vi "Initialize.vi"(8 "error in (no error)":errorcluster, 11 "State in":T1={"State"=enum."Idle", "Start Time"=timestamp(0 s since 1904-01-01), "Configuration"={"Cycle Period"=0.0, "Ismatech"={"VISA resource name"="", "Simulated?"=FALSE, "Pump Number"=1.0, "Reverse?"=FALSE}, "Masterflex"={"VISA resource name"="", "Simulated?"=FALSE, "Pump Number"=1.0, "Reverse?"=FALSE}, "Manual Entry"=0.0, "VICI Settings"={"VISA resource name"="", "Simulated?"=FALSE, "Pump Letter"="", "Reverse?"=FALSE}, "Output Device"=enum."Ismatec ISM 831C", "Tacmina Settings"={"Analog DAQ Task"="", "Digital DAQ Task"=""}, "KNF SIMDOS Settings"={"VISA resource name"="", "Simulated?"=TRUE}, "ASIA Pump C"={"ASIA Pump #"=0, "channel"=0, "Simulated"=FALSE}, "FLOM Settings"={"VISA resource name"="", "Simulated?"=TRUE, "Pump Number"=0.0}, "Pump Calibration File"=path "", "Calibration Slope"=0.0, "Calibration Y Intercept"=0.0, "Pump Cal Enum"=0, "SSI PR Settings"={"VISA resource name"="", "Simulated?"=FALSE}}, "Current Time"=timestamp(0 s since 1904-01-01), "First Iteration"=FALSE, "Data"={"Pump Speed"=0.0, "Pump Pressure"=0.0, "Pump Flow"=0.0}, "Process Name"="", "Pump On?"=enum."Off", "Output Error"=FALSE, "Log Started"=FALSE, "Overpressure Alarming"=FALSE} {"Configuration"."ASIA Pump C"."channel" min=0 max=1 step=1; "Configuration"."Masterflex"."Pump Number" min=1.0 max=20.0 step=1.0; "Configuration"."Ismatech"."Pump Number" min=1.0 max=20.0 step=1.0}) -> (0 "error out":errorcluster, 1 "Initialized":bool, 3 "State out":T1={"State"=enum."Idle", "Start Time"=timestamp(0 s since 1904-01-01), "Configuration"={"Cycle Period"=0.0, "Ismatech"={"VISA resource name"="", "Simulated?"=FALSE, "Pump Number"=1.0, "Reverse?"=FALSE}, "Masterflex"={"VISA resource name"="", "Simulated?"=FALSE, "Pump Number"=1.0, "Reverse?"=FALSE}, "Manual Entry"=0.0, "VICI Settings"={"VISA resource name"="", "Simulated?"=FALSE, "Pump Letter"="", "Reverse?"=FALSE}, "Output Device"=enum."Ismatec ISM 831C", "Tacmina Settings"={"Analog DAQ Task"="", "Digital DAQ Task"=""}, "KNF SIMDOS Settings"={"VISA resource name"="", "Simulated?"=TRUE}, "ASIA Pump C"={"ASIA Pump #"=0, "channel"=0, "Simulated"=FALSE}, "FLOM Settings"={"VISA resource name"="", "Simulated?"=TRUE, "Pump Number"=0.0}, "Pump Calibration File"=path "", "Calibration Slope"=0.0, "Calibration Y Intercept"=0.0, "Pump Cal Enum"=0, "SSI PR Settings"={"VISA resource name"="", "Simulated?"=FALSE}}, "Current Time"=timestamp(0 s since 1904-01-01), "First Iteration"=FALSE, "Data"={"Pump Speed"=0.0, "Pump Pressure"=0.0, "Pump Flow"=0.0}, "Process Name"="", "Pump On?"=enum."Off", "Output Error"=FALSE, "Log Started"=FALSE, "Overpressure Alarming"=FALSE} {"Configuration"."ASIA Pump C"."channel" min=0 max=1 step=1; "Configuration"."Masterflex"."Pump Number" min=1.0 max=20.0 step=1.0; "Configuration"."Ismatech"."Pump Number" min=1.0 max=20.0 step=1.0})   [LabVIEW 2018, in "Pump Module.lvlib" / "Pump Module Engine.lvlib"]
uses:
  Pump Module Engine.lvlib
  State Cluster.ctl
  State Enum.ctl
  Pump Module Settings Cluster.ctl
  Ismatec ISM 831C/Controls/Ismatech Settings Cluster.ctl
  Masterflex 7550-30/Controls/Settings Cluster.ctl
  VICI M50 Party Mode/Settings Cluster.ctl
  Measure Instrument/PID 2 Output Enum.ctl
  Tacmina QI/Tacmina QI DAQ Setting.ctl
  KNF Pump/Settings Cluster plus SIMDOS.ctl
  ASIA Pump/Pump Settings.ctl
  FLOM Pump/Settings Cluster.ctl
  SSI PR Class/SSI PR Settings Cluster.ctl
  Tag VIs/Tag FGV Operation Enum.ctl
  Shared Variables/Dynamic Shared Variables.lvlib
  SSI PR Class/SSI PR Pump.lvlib
  FLOM Pump/FLOM Pump.lvlib
  ASIA Pump.lvlib
  KNF Pump/KNF SIMDOS.lvlib
  Tacmina QI/Tacmina QI.lvlib
  VICI M50 Party Mode/VICI M6 M50 Party Mode.lvlib
  Ismatec ISM 831C/Ismatec ISM 831C.lvlib
  Masterflex 7550-30/Masterflex 7550-30.lvlib
  Pump Module.lvlib
panel:
  # "Output Instruments"
  # "Output Instruments"
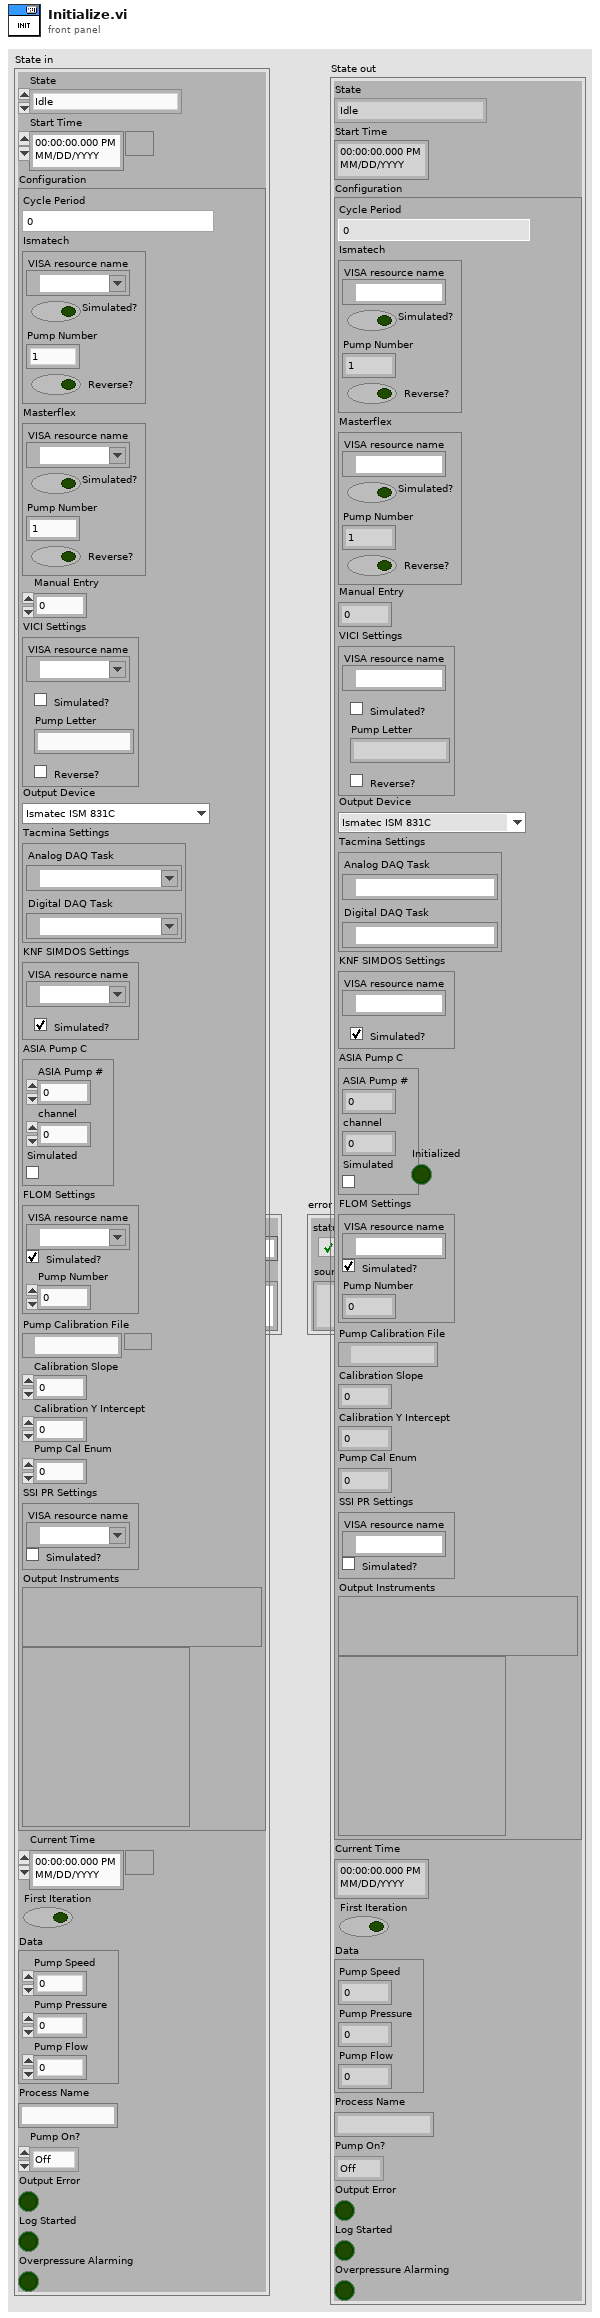
[diagram p1: front panel]
types:
  T1 = typedef "Pump Module.lvlib/Pump Module Engine.lvlib/State Cluster.ctl" = cluster{"State":T2, "Start Time":timestamp, "Configuration":T3, "Current Time":timestamp, "First Iteration":bool, "Data":cluster{"Pump Speed":dbl, "Pump Pressure":dbl, "Pump Flow":dbl}, "Process Name":string, "Pump On?":enum16{"Off", "On", "Not Initialized"}, "Output Error":bool, "Log Started":bool, "Overpressure Alarming":bool}
  T2 = typedef "Pump Module.lvlib/Pump Module Engine.lvlib/State Enum.ctl" = enum16{"Measuring", "Idle", "Paused"}
  T3 = typedef "Pump Module.lvlib/Pump Module Settings Cluster.ctl" = cluster{"Cycle Period":dbl, "Ismatech":T4, "Masterflex":T5, "Manual Entry":dbl, "VICI Settings":T6, "Output Device":T7, "Tacmina Settings":T8, "KNF SIMDOS Settings":T9, "ASIA Pump C":T10, "FLOM Settings":T11, "Pump Calibration File":path, "Calibration Slope":dbl, "Calibration Y Intercept":dbl, "Pump Cal Enum":u16, "SSI PR Settings":T12}
  T4 = typedef "Ismatec ISM 831C.lvlib/Ismatech Settings Cluster.ctl" = cluster{"VISA resource name":refnum<visa-resource-name>, "Simulated?":bool, "Pump Number":dbl, "Reverse?":bool}
  T5 = typedef "Masterflex 7550-30.lvlib/Settings Cluster.ctl" = cluster{"VISA resource name":refnum<visa-resource-name>, "Simulated?":bool, "Pump Number":dbl, "Reverse?":bool}
  T6 = typedef "VICI M6 M50 Party Mode.lvlib/Settings Cluster.ctl" = cluster{"VISA resource name":refnum<visa-resource-name>, "Simulated?":bool, "Pump Letter":string, "Reverse?":bool}
  T7 = typedef "PID 2 Output Enum.ctl" = enum16{"Default", "Ismatec ISM 831C", "Masterflex 7550-30", "VICI", "Tacmina QI", "KNF SIMDOS", "ASIA Type C", "FLOM UI-22-11", "SSI PR"}
  T8 = typedef "Tacmina QI.lvlib/Tacmina QI DAQ Setting.ctl" = cluster{"Analog DAQ Task":refnum<k21>, "Digital DAQ Task":refnum<k21>}
  T9 = typedef "KNF SIMDOS.lvlib/Settings Cluster plus SIMDOS.ctl" = cluster{"VISA resource name":refnum<visa-resource-name>, "Simulated?":bool}
  T10 = typedef "ASIA Pump.lvlib/Pump Settings.ctl" = cluster{"ASIA Pump #":i32, "channel":i32, "Simulated":bool}
  T11 = typedef "FLOM Pump.lvlib/Settings Cluster.ctl" = cluster{"VISA resource name":refnum<visa-resource-name>, "Simulated?":bool, "Pump Number":dbl}
  T12 = typedef "SSI PR Pump.lvlib/SSI PR Settings Cluster.ctl" = cluster{"VISA resource name":refnum<visa-resource-name>, "Simulated?":bool}
  T13 = cluster{"Output Device":T7, "Masterflex":T5, "Ismatech":T4, "VICI M50 Settings":T6, "Tacmina Settings":T8, "KNF SIMDOS Settings":T9, "ASIA Pump C":T10, "FLOM Settings":T11, "SSI PR Settings":T12}
  T14 = typedef "Tag FGV Operation Enum.ctl" = enum16{"Init", "Set Notification Queue", "Create Tag", "Commit", "Write Tag (Numeric)", "Write Tag (Boolean)", "Read All Tags", "Read One Tag", "Delete Tag Category", "Set Alarm Parameters (Numeric)", "Set Alarm Parameters (Boolean)", "Enable All Alarms", "Disable All Alarms", "Delete All Tags", "Read Alarms", "Ack Alarm", "Read Alarm Parameters (Numeric)", "Read Alarm Parameters (Boolean)"}
  T15 = typedef "Pump Module.lvlib/Pump Module Tag Names Cluster.ctl" = cluster{"Pump Speed":string, "Pump Flow":string, "Pump Pressure":string, "Output Device Tag":string, "Overpressure Tag":string}
  T16 = typedef "Pump Module.lvlib/Pump Settings Cluster.ctl" = cluster{"Output Device":T7, "Masterflex":T5, "Ismatech":T4, "VICI Settings":T6, "Tacmina Settings":T8, "KNF SIMDOS Settings":T9, "ASIA Pump C":T10, "FLOM Settings":T11, "SSI PR Settings":T12}
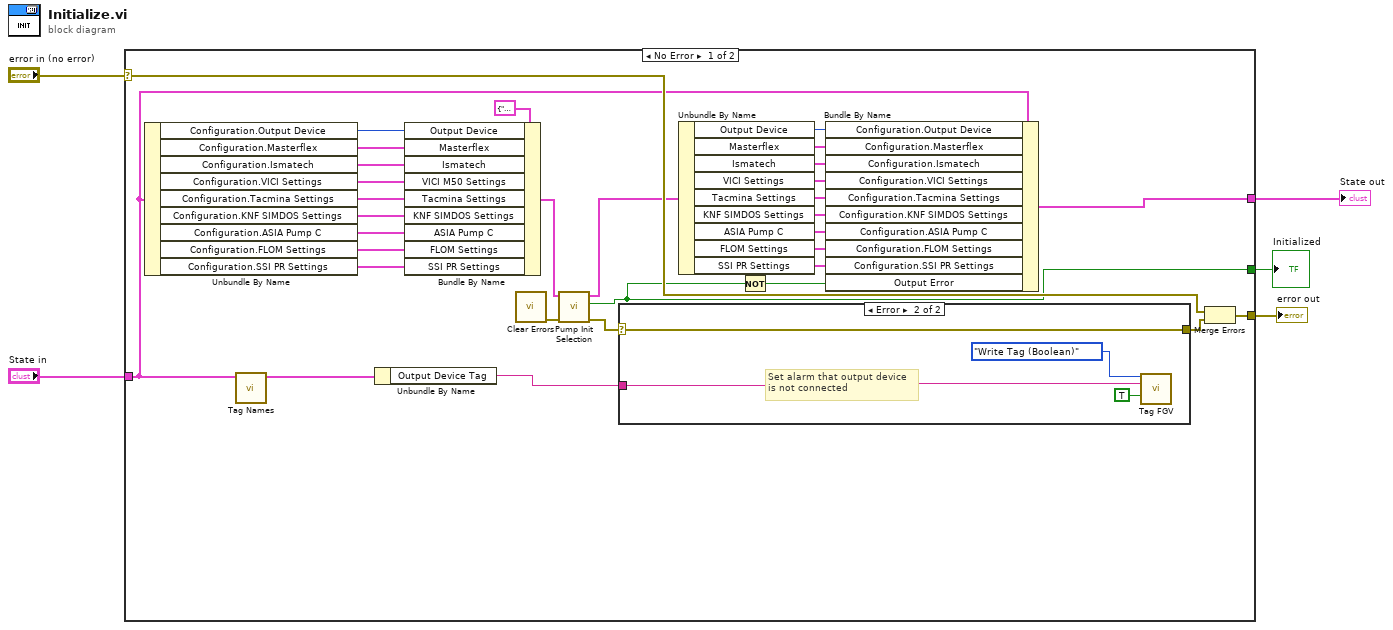
[diagram p0: block diagram]
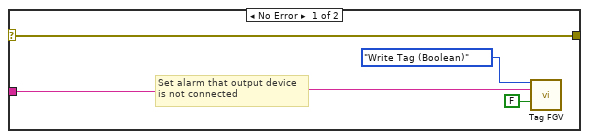
[diagram p2: hidden frame]
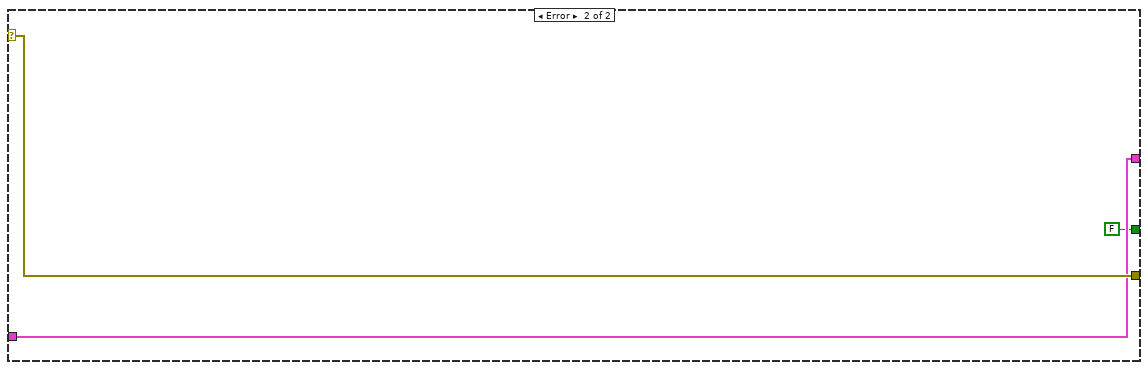
[diagram p3: hidden frame]
diagram:
  n1 = case shown="No Error" "error in (no error)" {
    selector: "error in (no error)" -> [w32 w48]
    tunnel: [w36 w48] -> w4
    tunnel: "State in" -> [w19 w47]
    tunnel: [w18 w47] -> w2
    tunnel: [w6 FALSE ("Initialized")] -> w1
    frame No Error {
      n2 = Unbundle By Name(w19) -> ("Configuration.Output Device"=w29:T7, "Configuration.Masterflex"=w28:T5, "Configuration.Ismatech"=w27:T4, "Configuration.VICI Settings"=w26:T6, "Configuration.Tacmina Settings"=w25:T8, "Configuration.KNF SIMDOS Settings"=w24:T9, "Configuration.ASIA Pump C"=w23:T10, "Configuration.FLOM Settings"=w22:T11, "Configuration.SSI PR Settings"=w21:T12)
      n3 = call "Tag Names.vi"("State In"=w19) -> ("Pump Module Tag Names"=w31:T15)  [unwired: 8 in, 2 out]
      n4 = Unbundle By Name(w31) -> ("Output Device Tag"=w33:string)
      n5 = Bundle By Name(cluster=T13 {"Output Device"=enum."Default", "Masterflex"={"VISA resource name"="", "Simulated?"=FALSE, "Pump Number"=0.0, "Reverse?"=FALSE}, "Ismatech"={"VISA resource name"="", "Simulated?"=FALSE, "Pump Number"=0.0, "Reverse?"=FALSE}, "VICI M50 Settings"={"VISA resource name"="", "Simulated?"=FALSE, "Pump Letter"="", "Reverse?"=FALSE}, "Tacmina Settings"={"Analog DAQ Task"="", "Digital DAQ Task"=""}, "KNF SIMDOS Settings"={"VISA resource name"="", "Simulated?"=FALSE}, "ASIA Pump C"={"ASIA Pump #"=0, "channel"=0, "Simulated"=FALSE}, "FLOM Settings"={"VISA resource name"="", "Simulated?"=FALSE, "Pump Number"=0.0}, "SSI PR Settings"={"VISA resource name"="", "Simulated?"=FALSE}} ("Pump Settings In"), "Output Device"=w29, "Masterflex"=w28, "Ismatech"=w27, "VICI M50 Settings"=w26, "Tacmina Settings"=w25, "KNF SIMDOS Settings"=w24, "ASIA Pump C"=w23, "FLOM Settings"=w22, "SSI PR Settings"=w21) -> (w20:T13)
      n6 = call <vilib>:"Clear Errors.vi"() -> ("error out"=w37:errorcluster)  [unwired: 6 in, 1 out]
      n7 = call "Pump Init Selection.vi"("error in (no error)"=w37, "Pump Settings In"=w20) -> ("error out"=w35:errorcluster, "Initialized"=w6:bool, "Pump Settings Out"=w17:T16)  [unwired: 7 in]
      n8 = case shown="Error" w35 {
        selector: w35 -> [w41 w45]
        tunnel: [w41 w45] -> w34
        tunnel: w33 -> [w38 w44]
        frame No Error {
          # "Set alarm that output device\nis not connected"
          n9 = call "Tag FGV.vi"("Operation"=Tag_FGV_Operation_Enum."Write Tag (Boolean)", "Tag Name"=w38, "Data"=FALSE) -> ()  [unwired: 5 in, 8 out]
        }
        frame Error {
          # "Set alarm that output device\nis not connected"
          n10 = call "Tag FGV.vi"("Operation"=Tag_FGV_Operation_Enum."Write Tag (Boolean)", "Tag Name"=w44, "Data"=TRUE) -> ()  [unwired: 5 in, 8 out]
        }
      }
      n11 = Unbundle By Name(w17) -> ("Output Device"=w16:T7, "Masterflex"=w15:T5, "Ismatech"=w14:T4, "VICI Settings"=w13:T6, "Tacmina Settings"=w12:T8, "KNF SIMDOS Settings"=w11:T9, "ASIA Pump C"=w10:T10, "FLOM Settings"=w9:T11, "SSI PR Settings"=w8:T12)
      n12 = Not(x=w6) -> (.not. x?=w7:bool)
      n13 = Bundle By Name(cluster=w19, "Configuration.Output Device"=w16, "Configuration.Masterflex"=w15, "Configuration.Ismatech"=w14, "Configuration.VICI Settings"=w13, "Configuration.Tacmina Settings"=w12, "Configuration.KNF SIMDOS Settings"=w11, "Configuration.ASIA Pump C"=w10, "Configuration.FLOM Settings"=w9, "Configuration.SSI PR Settings"=w8, "Output Error"=w7) -> (w18:T1)
      n14 = Merge Errors(w32, w34) -> (w36:errorcluster)
    }
    frame Error {
    }
  }
  "error out" <- w4
  "State out" <- w2
  "Initialized" <- w1
